vi "当前路径选择.vi"(1 "本应用程序":refnum<vi>) -> (0 "当前路径":path)   [LabVIEW 2015]
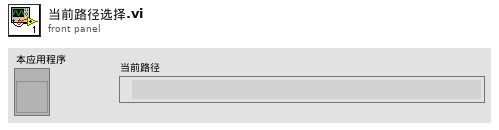
[diagram p1: front panel]
types:
  T1 = enum32{"invalid app kind", "Development System", "Run Time System", "Student Edition", "Embedded LabVIEW", "Evaluation", "Custom"}
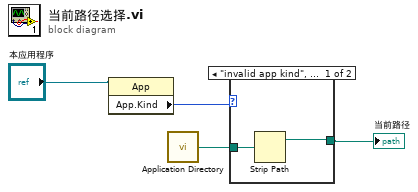
[diagram p0: block diagram]
diagram:
  n1 = property class="App"(reference="本应用程序") -> ("App.Kind"=w3:T1)  [unwired: 1 in, 2 out]
  n2 = call <vilib>:"Application Directory.vi"() -> ("Application Directory"=w4:path)
  n3 = case shown="\"invalid app kind\", 默认" w3 {
    tunnel: [w5 w7] -> w1
    tunnel: w4 -> [w6 w7]
    frame "invalid app kind", Default {
      n4 = Strip Path(path=w6) -> (stripped path=w5:path)  [unwired: 1 out]
    }
    frame "Development System" {
    }
  }
  "当前路径" <- w1
